vi "Write Tick Colors.vi"(5 "Tick Colors":T1, 9 "Scale in":refnum<class "Scale.lvclass">) -> (3 "Scale out":refnum<class "Scale.lvclass">)   [LabVIEW 2014, in "Scale.lvclass"]
uses:
  Scale.lvclass
  <vilib>/Utility/miscctls.llb/LVTickColorsTypeDef.ctl
  Scale.lvclass/Scale.ctl
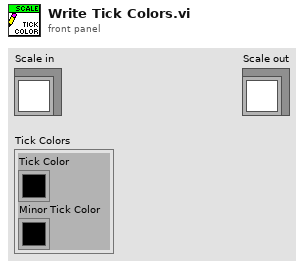
[diagram p1: front panel]
types:
  T1 = typedef "LVTickColorsTypeDef.ctl" = cluster{"Tick Color":u32, "Minor Tick Color":u32}
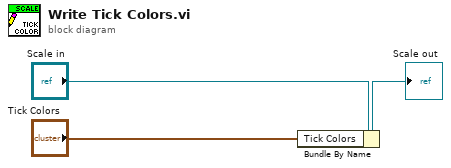
[diagram p0: block diagram]
diagram:
  n1 = Bundle By Name(cluster="Scale in", "Tick Colors"="Tick Colors") -> (→"Scale out":refnum<class "Scale.lvclass">)
